vi "Rings In A Cluster.vi"(10 "String":string, 11 "Cluster":T4={"Numeric"=0.0, "Inner Cluster - Level 1"={"String"="", "Numbers Enum"=enum."Two", "Boolean"=FALSE, "Cluster"={"Numeric"=0.0, "String"="", "Text Ring"=3}, "Array Of Enums"=[11, 33, 125]}} {"Inner Cluster - Level 1"."Array Of Enums" items=["Menu Option 11"=11, "Menu Option 45"=45, "Menu Option 33"=33, "Menu Option 75"=75, "Menu Option 125"=125]; "Inner Cluster - Level 1"."Cluster"."Text Ring" items=["Text Value 0", "Text Value 1", "Text Value 2", "Text Value 3", "Text Value 5", "Text Value 6"]}) -> ()   [LabVIEW 2012]
uses:
  EnumTypeDefControl.ctl
  TextRingTypeDefControl.ctl
  MenuRingTypeDefControl.ctl
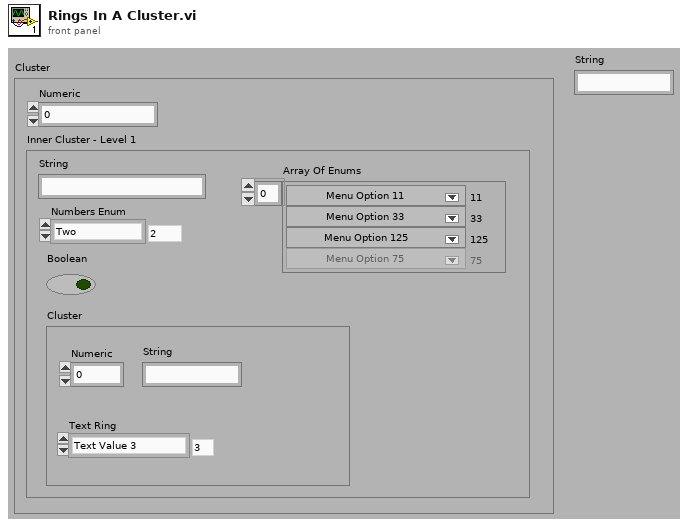
[diagram p1: front panel]
types:
  T1 = typedef "EnumTypeDefControl.ctl" = enum8{"Zero", "One", "Two", "Three", "Four", "Five"}
  T2 = typedef "TextRingTypeDefControl.ctl" = u16
  T3 = typedef "MenuRingTypeDefControl.ctl" = u32
  T4 = cluster{"Numeric":dbl, "Inner Cluster - Level 1":cluster{"String":string, "Numbers Enum":T1, "Boolean":bool, "Cluster":cluster{"Numeric":dbl, "String":string, "Text Ring":T2}, "Array Of Enums":T3[]}}
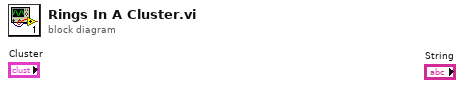
[diagram p0: block diagram]
diagram:
